vi "LowPassFilterOma.vi"(10 "Numeric":dbl, 11 "Numeric 2":dbl) -> (2 "Filtered x":dbl, 3 "Filtered x 2":dbl)   [LabVIEW 2016]
uses:
  <vilib>/ptbypt/NI_PtbyPt.lvlib
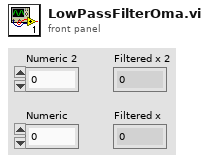
[diagram p1: front panel]
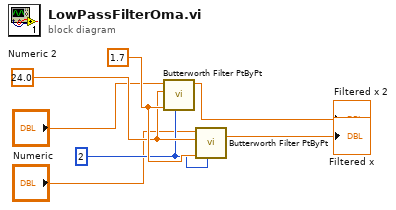
[diagram p0: block diagram]
diagram:
  w7 = 1.7 ("low cutoff freq: fl")
  w6 = 24.0 ("sampling freq: fs")
  w5 = 2 ("order")
  n1 = call <vilib>:"Butterworth Filter PtByPt.vi"("order"=w5, "low cutoff freq: fl"=w7, "sampling freq: fs"=w6, "x"="Numeric 2") -> ("Filtered x"=→"Filtered x 2":dbl)  [unwired: 5 in, 1 out]
  n2 = call <vilib>:"Butterworth Filter PtByPt.vi"("order"=w5, "low cutoff freq: fl"=w7, "sampling freq: fs"=w6, "x"="Numeric") -> ("Filtered x"=→"Filtered x":dbl)  [unwired: 5 in, 1 out]
